vi "maska.vi"() -> ()   [LabVIEW 2023]
panel:
  out "Tablica maskowana":bool[](array[boolean])
  out "Maska":bool[](array[boolean])
  out "Tablica":bool[](array[boolean])
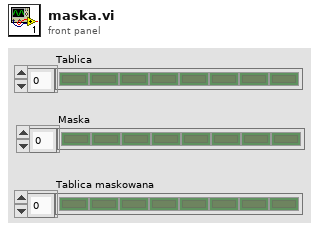
[diagram p1: front panel]
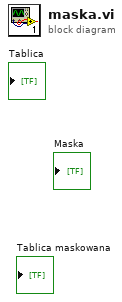
[diagram p0: block diagram]
diagram:
